vi "Initialize Step.vi"(8 "error in (no error)":errorcluster, 11 "Base Step in":refnum<class "Base Step.lvclass">) -> (0 "error out":errorcluster, 3 "Base Step out":refnum<class "Base Step.lvclass">)   [LabVIEW 2024, in "Ramses Sequencer.lvlib" / "Base Step.lvclass"]
uses:
  Base Step.lvclass
  Typedefs/Step State.ctl
  Base Step.lvclass/Base Step.ctl
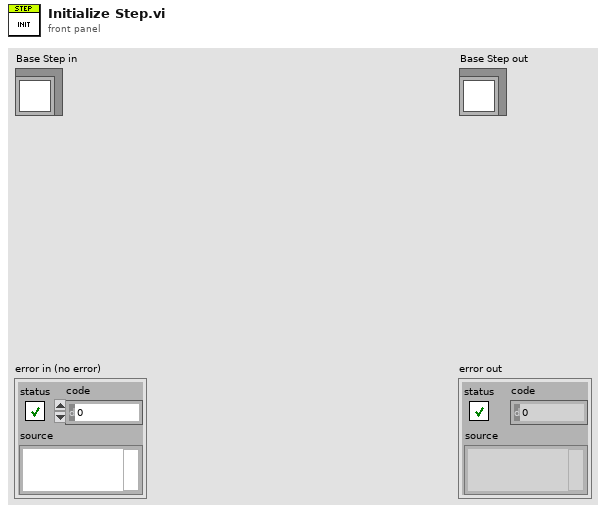
[diagram p1: front panel]
types:
  T1 = typedef "Ramses Sequencer.lvlib/Base Step.lvclass/Step State.ctl" = cluster{"Result":string, "Status":string, "Enabled":bool, "Upper":string, "Target":string, "Lower":string, "Value":string}
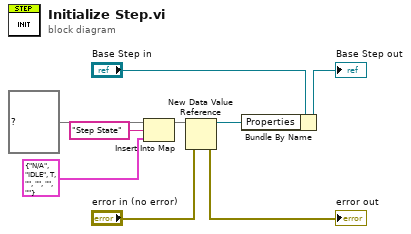
[diagram p0: block diagram]
diagram:
  n1 = Insert Into Map(map in=map{string, variant} {} ("Properties"), key="Step State", value=T1 {"Result"="N/A", "Status"="IDLE", "Enabled"=TRUE, "Upper"="", "Target"="", "Lower"="", "Value"=""} ("Step State")) -> (map out=w8:map{string, variant})  [unwired: 2 out]
  n2 = New Data Value Reference(data value=w8, error in="error in (no error)") -> (data value reference=w4:refnum<data-value>, error out=→"error out":errorcluster)
  n3 = Bundle By Name(cluster="Base Step in", "Properties"=w4) -> (→"Base Step out":refnum<class "Base Step.lvclass">)
